vi "Main RT.vi"() -> ()   [LabVIEW 2014]
uses:
  Controls/RT State.ctl
  Controls/Current Limit Parameters.ctl
  Controls/ES System Data.ctl
  Controls/StringSelector.ctl
  Controls/FPGA Data.ctl
  Controls/ES String Array.ctl
  Controls/ES String Data.ctl
  Controls/PC Data.ctl
  Controls/MicroZed Config Op Mode.ctl
  Controls/MicroZed Config.ctl
  Controls/Gen Data.ctl
  Controls/Current Limit Output.ctl
  <vilib>/Modbus/subvis/Modbus API/Modbus API.lvclass/Modbus API.ctl
  <vilib>/Modbus/subvis/Transmission Data Unit (ADU)/Transmission Data Unit/Transmission Data Unit.lvclass/Transmission Data Unit.ctl
  <vilib>/Modbus/master/Set Unit ID.vi
  <vilib>/Modbus/master/Data Access/Unit ID/Set Unit ID Property.vi
  <vilib>/Modbus/subvis/Transmission Data Unit (ADU)/Transmission Data Unit/Data Access/Unit ID/Write Unit ID.vi
  <vilib>/Modbus/subvis/Modbus API/Read Transmission Data Unit.vi
  <vilib>/Modbus/subvis/Modbus API/Write Transmission Data Unit.vi
  <vilib>/FPGAPlugInAG/cRIO-9068/niLvFpga_Open_cRIO-9068.vi
  <vilib>/rvi/interface/common/dynamic/niFpgaDynamicAddResources.vi
  <vilib>/FPGAPlugInAG/Dynamic/niLvFpga_Reset_Dynamic.vi
  <vilib>/FPGAPlugInAG/Dynamic/niLvFpga_Run_Dynamic.vi
  <vilib>/Utility/error.llb/Error Cluster From Error Code.vi
  <vilib>/rvi/errors/niLvFpgaAdjustHostInterfaceError.vi
  <vilib>/Modbus/master/Create Master Instance.vi
  <vilib>/Modbus/master/Create Master Instance (TCP).vi
  <vilib>/Modbus/master/Set Timeouts.vi
  GenErrorParse.vi
  32Bit Two Complement.vi
  16Bit Two Complement.vi
  <vilib>/FPGAPlugInAG/Dynamic/niLvFpga_Close_Dynamic.vi
  <vilib>/rvi/interface/nirviOpenFPGA/nirviOpenFPGA.xnode
  Builds/FPGA Bitfiles/FPGA NIGHTVISION.lvbitx
  <vilib>/rvi/interface/nirviMethod/nirviMethod.xnode
  <vilib>/rvi/interface/nirviReadWriteControl/nirviReadWriteControl.xnode
  <vilib>/Modbus/master/Modbus Master.lvclass
  <vilib>/Modbus/subvis/Transmission Data Unit (ADU)/Transmission Data Unit/Transmission Data Unit.lvclass
  <vilib>/rvi/interface/nirviCloseFPGA/nirviCloseFPGA.xnode
  RT Watchdog/RT Watchdog.lvlib
  NiFpgaLv.dll
  <vilib>/rvi/interface/Simulation/niFpgaSimulationCallBeginRW.vi
  <vilib>/ptbypt/NI_PtbyPt.lvlib
panel:
  in  "PC CMD":bool=TRUE
  out "Charge Max SOC":sgl=55.0
  out "HVAC FB":bool
  out "HVAC CMD":bool=TRUE
  out "Contactor CMD FB":bool[](array[boolean])
  out "ES Cycle Count":dbl
  out "Write Data":string[](array[string])
  out "Read Data":string[](array[string])
  in  "Manual OLP":T1 {"Min Cell Voltage Actual Value" format="%#.2f"; "Max Cell Voltage Actual Value" format="%#.2f"}
  in  "Override?":bool
  out "First String Index":i32
  out "PC Count":i32
  out "Gen East Count":i32
  out "Gen West Count":i32
  out "ES Count":i32
  out "Generator ON East":bool=TRUE
  out "Generator ON West":bool=TRUE
  out "Gen Active":T2={"Warning"=FALSE, "System Fault"=FALSE, "Com Fault"=TRUE, "Alarms"=[], "ControllerMode"=0, "ActivePower(W)"=0, "ReactivePower(VAR)"=0, "PowerFactor"=0.0, "RunHours(hr)"=0.0, "Freq(Hz)"=0.0, "BattVoltage(V)"=0.0, "ApparentPower(VA)"=0, "FuelRate(L/H)"=0.0, "TotalFuel(L)"=0, "IsRunning"=FALSE} {"TotalFuel(L)" format="%.2f"; "FuelRate(L/H)" format="%.2f"; "ApparentPower(VA)" format="%.2f"; "BattVoltage(V)" format="%.2f"; "Freq(Hz)" format="%.2f"; "RunHours(hr)" format="%.2f"; "PowerFactor" format="%.2f"; "ReactivePower(VAR)" format="%.2f"; "ActivePower(W)" format="%.2f"}
  out "Gen Data East":T2={"Warning"=FALSE, "System Fault"=FALSE, "Com Fault"=TRUE, "Alarms"=[], "ControllerMode"=0, "ActivePower(W)"=0, "ReactivePower(VAR)"=0, "PowerFactor"=0.0, "RunHours(hr)"=0.0, "Freq(Hz)"=0.0, "BattVoltage(V)"=0.0, "ApparentPower(VA)"=0, "FuelRate(L/H)"=0.0, "TotalFuel(L)"=0, "IsRunning"=FALSE} {"TotalFuel(L)" format="%.2f"; "FuelRate(L/H)" format="%.2f"; "ApparentPower(VA)" format="%.2f"; "BattVoltage(V)" format="%.2f"; "Freq(Hz)" format="%.2f"; "RunHours(hr)" format="%.2f"; "PowerFactor" format="%.2f"; "ReactivePower(VAR)" format="%.2f"; "ActivePower(W)" format="%.2f"}
  out "Gen Data West":T2={"Warning"=FALSE, "System Fault"=FALSE, "Com Fault"=TRUE, "Alarms"=[], "ControllerMode"=0, "ActivePower(W)"=0, "ReactivePower(VAR)"=0, "PowerFactor"=0.0, "RunHours(hr)"=0.0, "Freq(Hz)"=0.0, "BattVoltage(V)"=0.0, "ApparentPower(VA)"=0, "FuelRate(L/H)"=0.0, "TotalFuel(L)"=0, "IsRunning"=FALSE} {"TotalFuel(L)" format="%.2f"; "FuelRate(L/H)" format="%.2f"; "ApparentPower(VA)" format="%.2f"; "BattVoltage(V)" format="%.2f"; "Freq(Hz)" format="%.2f"; "RunHours(hr)" format="%.2f"; "PowerFactor" format="%.2f"; "ReactivePower(VAR)" format="%.2f"; "ActivePower(W)" format="%.2f"}
  in  "Genset On":bool=TRUE
  out "Current Limit Output":T3
  in  "Automatic Start":bool
  in  "Clear Error":bool
  in  "PV Breaker":bool
  in  "SSG Breaker":bool
  in  "PC Config":T4={"AC Voltage SP"=0.0, "AC Current SP"=0.0, "Frequency SP"=60.0, "DC Voltage SP"=450.0, "Op Mode SP"=enum."Shutdown (Reset)", "Clear Faults SP"=0} {"Clear Faults SP" format="%01x"; "DC Voltage SP" min=300 max=550 format="%2.1f"; "Frequency SP" min=45 max=65 format="%2.1f"; "AC Current SP" min=-500 max=500 format="%2.1f"; "AC Voltage SP" min=0 max=132 format="%2.1f"}
  out "PC Data":T6={"AC Voltage- L1"=0.0, "AC Voltage - L2"=0.0, "AC Current - L1"=0.0, "AC Current - L2"=0.0, "Neutral Current"=0.0, "Temperature"=0.0, "AC Frequency"=0.0, "DC Voltage"=0.0, "AC Voltage SP"=0.0, "AC Current SP"=0.0, "Frequency SP"=0.0, "Op Mode SP"=enum."Shutdown (Reset)", "Clear Faults SP"=0, "PC Com Fault"=TRUE, "PC Fault"=FALSE, "DC Voltage SP"=0.0, "OP Mode FB"=enum."Shutdown (Reset)", "Contactor FB"=0, "Faults 1"=0, "Alarms 1"=0, "Faults 2"=0, "Alarms 2"=0, "PC Alarm"=FALSE, "Version"=0} {"Alarms 2" format="%016b"; "Faults 2" format="%016b"; "Alarms 1" format="%016b"; "Faults 1" format="%016b"; "Contactor FB" format="%.0b"; "DC Voltage SP" format="%2.1f"; "Clear Faults SP" format="%.0b"; "Neutral Current" format="%2.1f"; "AC Current - L2" format="%2.1f"; "AC Voltage - L2" format="%2.1f"; "Temperature" format="%2.1f"; "DC Voltage" format="%2.1f"; "AC Current SP" format="%2.1f"; "AC Voltage SP" format="%2.1f"; "Frequency SP" format="%2.1f"; "AC Frequency" format="%2.1f"; "AC Current - L1" format="%2.1f"; "AC Voltage- L1" format="%2.1f"}
  in  "ES ON Array":bool[](array[boolean])
  out "ES String Data":T7
  out "FPGA Data":T9 {"SSG Active Current" format="%2.1f"; "PV Reactive Power (L1)" format="%2.1f"; "PV Reactive Power (L2)" format="%2.1f"; "PV Total Reactive Power" format="%2.1f"; "Gen Reactive Power (L1)" format="%2.1f"; "Gen Reactive Power (L2)" format="%2.1f"; "Gen Total Reactive Power" format="%2.1f"; "SSG Reactive Power (L1)" format="%2.1f"; "SSG Reactive Power (L2)" format="%2.1f"; "SSG Total Reactive Power" format="%2.1f"; "PV Total Current" format="%2.1f"; "PV Total Voltage" format="%2.1f"; "PV Active Power (L1)" format="%2.1f"; "PV Active Power (L2)" format="%2.1f"; "PV App Power (L1)" format="%2.1f"; "PV App Power (L2)" format="%2.1f"; "PV Total Active Power" format="%2.1f"; "PV Total App Power" format="%2.1f"; "PV Arms (L1)" format="%2.1f"; "PV Arms (L2)" format="%2.1f"; "PV Vrms (L1)" format="%2.1f"; "PV Vrms (L2)" format="%2.1f"; "Gen Total Current" format="%2.1f"; "SSG Total Current" format="%2.1f"; "Gen Total Voltage" format="%2.1f"; "SSG Total Voltage" format="%2.1f"; "Gen Active Power (L1)" format="%2.1f"; "Gen Active Power (L2)" format="%2.1f"; "SSG Active Power (L1)" format="%2.1f"; "SSG Active Power (L2)" format="%2.1f"; "Gen App Power (L1)" format="%2.1f"; "Gen App Power (L2)" format="%2.1f"; "SSG App Power (L1)" format="%2.1f"; "SSG App Power (L2)" format="%2.1f"; "Gen Total Active Power" format="%2.1f"; "Gen Total App Power" format="%2.1f"; "Gen Arms (L1)" format="%2.1f"; "Gen Arms (L2)" format="%2.1f"; "Gen Vrms (L1)" format="%2.1f"; "Gen Vrms (L2)" format="%2.1f"; "SSG Total Active Power" format="%2.1f"; "SSG Total App Power" format="%2.1f"; "SSG Arms (L1)" format="%2.1f"; "SSG Arms (L2)" format="%2.1f"; "SSG Vrms (L1)" format="%2.1f"; "SSG Vrms (L2)" format="%2.1f"}
  out "ES System Data":T10={"Voltage"=0.0, "Current"=0.0, "SOC Avg"=0.0, "Faults"=0, "Alarms"=0, "# Strings"=0, "Max Temp"=0, "Min Temp"=0, "Max Cell Voltage"=0.0, "Min Cell Voltage"=0.0, "Energy Capacity"=0.0, "Energy Remaining"=0.0, "SOC Min"=0.0, "SOC Max"=0.0, "ES Fault"=FALSE, "String Select"=enum."3 Strings", "ES Com Fault"=TRUE, "SOH Avg"=0.0}
  out "Current Limit Parameters":T1 {"Min Cell Voltage Actual Value" format="%#.2f"; "Max Cell Voltage Actual Value" format="%#.2f"}
  out "Real Time State":T12
  in  "stop":bool
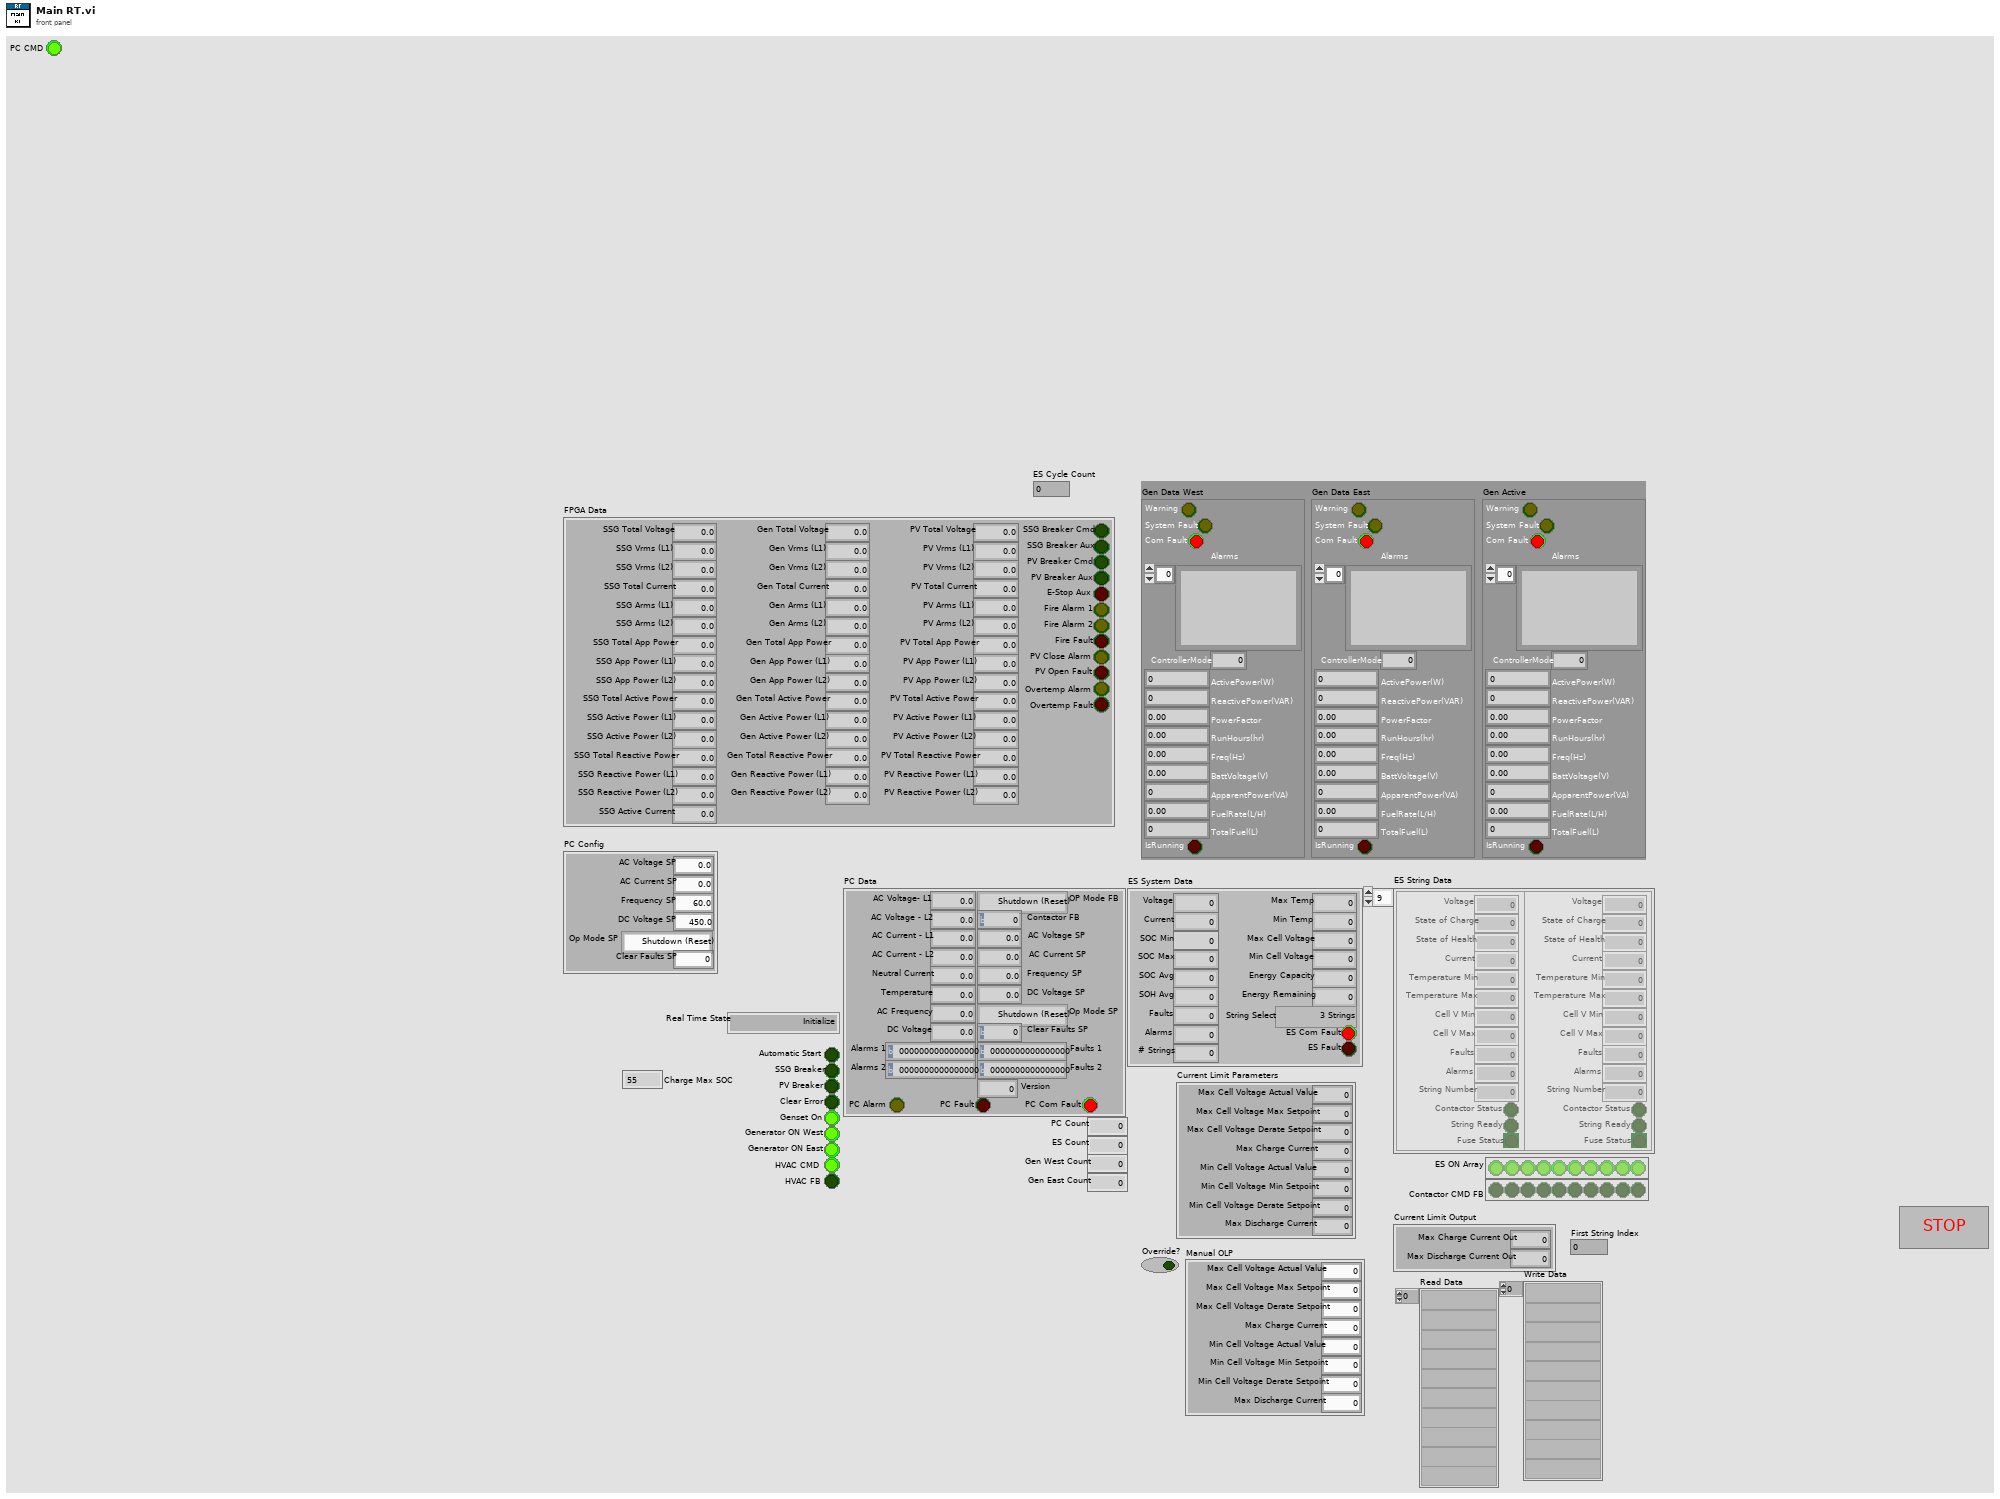
[diagram p1: front panel]
types:
  T1 = typedef "Current Limit Parameters.ctl" = cluster{"Max Cell Voltage Max Setpoint":dbl, "Max Cell Voltage Actual Value":dbl, "Max Cell Voltage Derate Setpoint":dbl, "Max Charge Current":dbl, "Min Cell Voltage Min Setpoint":dbl, "Min Cell Voltage Actual Value":dbl, "Min Cell Voltage Derate Setpoint":dbl, "Max Discharge Current":dbl}
  T2 = typedef "Gen Data.ctl" = cluster{"Warning":bool, "System Fault":bool, "Com Fault":bool, "Alarms":string[], "ControllerMode":u16, "ActivePower(W)":i32, "ReactivePower(VAR)":i32, "PowerFactor":dbl, "RunHours(hr)":dbl, "Freq(Hz)":dbl, "BattVoltage(V)":dbl, "ApparentPower(VA)":i32, "FuelRate(L/H)":dbl, "TotalFuel(L)":u32, "IsRunning":bool}
  T3 = typedef "Current Limit Output.ctl" = cluster{"Max Charge Current Out":dbl, "Max Discharge Current Out":dbl}
  T4 = typedef "MicroZed Config.ctl" = cluster{"AC Voltage SP":sgl, "AC Current SP":sgl, "Frequency SP":sgl, "DC Voltage SP":sgl, "Op Mode SP":T5, "Clear Faults SP":i16}
  T5 = typedef "MicroZed Config Op Mode.ctl" = enum16{"Shutdown (Reset)", "Startup", "Idle", "Voltage Mode", "Current Mode", "Fault", "OL Voltage (Debug)", "No Data"}
  T6 = typedef "PC Data.ctl" = cluster{"AC Voltage- L1":dbl, "AC Voltage - L2":dbl, "AC Current - L1":dbl, "AC Current - L2":dbl, "Neutral Current":dbl, "Temperature":dbl, "AC Frequency":dbl, "DC Voltage":dbl, "AC Voltage SP":dbl, "AC Current SP":dbl, "Frequency SP":dbl, "Op Mode SP":T5, "Clear Faults SP":u16, "PC Com Fault":bool, "PC Fault":bool, "DC Voltage SP":dbl, "OP Mode FB":T5, "Contactor FB":u16, "Faults 1":u16, "Alarms 1":u16, "Faults 2":u16, "Alarms 2":u16, "PC Alarm":bool, "Version":u16}
  T7 = typedef "ES String Array.ctl" = T8[]
  T8 = typedef "ES String Data.ctl" = cluster{"Voltage":sgl, "State of Charge":sgl, "Current":sgl, "Temperature Min":i16, "Temperature Max":i16, "Faults":u16, "Alarms":u16, "String Number":u16, "Contactor Status":bool, "String Ready":bool, "Fuse Status":bool, "Cell V Max":dbl, "Cell V Min":dbl, "State of Health":sgl}
  T9 = typedef "FPGA Data.ctl" = cluster{"Gen Total Voltage":dbl, "Gen Vrms (L1)":dbl, "Gen Vrms (L2)":dbl, "Gen Total Current":dbl, "Gen Arms (L1)":dbl, "Gen Arms (L2)":dbl, "Gen Total App Power":dbl, "Gen App Power (L1)":dbl, "Gen App Power (L2)":dbl, "Gen Total Active Power":dbl, "Gen Active Power (L1)":dbl, "Gen Active Power (L2)":dbl, "Gen Total Reactive Power":dbl, "Gen Reactive Power (L1)":dbl, "Gen Reactive Power (L2)":dbl, "SSG Total Voltage":dbl, "SSG Vrms (L1)":dbl, "SSG Vrms (L2)":dbl, "SSG Total Current":dbl, "SSG Arms (L1)":dbl, "SSG Arms (L2)":dbl, "SSG Total App Power":dbl, "SSG App Power (L1)":dbl, "SSG App Power (L2)":dbl, "SSG Total Active Power":dbl, "SSG Active Power (L1)":dbl, "SSG Active Power (L2)":dbl, "SSG Total Reactive Power":dbl, "SSG Reactive Power (L1)":dbl, "SSG Reactive Power (L2)":dbl, "PV Total Voltage":dbl, "PV Vrms (L1)":dbl, "PV Vrms (L2)":dbl, "PV Total Current":dbl, "PV Arms (L1)":dbl, "PV Arms (L2)":dbl, "PV Total App Power":dbl, "PV App Power (L1)":dbl, "PV App Power (L2)":dbl, "PV Total Active Power":dbl, "PV Active Power (L1)":dbl, "PV Active Power (L2)":dbl, "PV Total Reactive Power":dbl, "PV Reactive Power (L1)":dbl, "PV Reactive Power (L2)":dbl, "SSG Breaker Cmd":bool, "SSG Breaker Aux":bool, "PV Breaker Cmd":bool, "PV Breaker Aux":bool, "E-Stop Aux":bool, "Fire Alarm 1":bool, "Fire Alarm 2":bool, "Fire Fault":bool, "PV Close Alarm":bool, "SSG Active Current":dbl, "Overtemp Alarm":bool, "Overtemp Fault":bool, "PV Open Fault":bool}
  T10 = typedef "ES System Data.ctl" = cluster{"Voltage":sgl, "Current":sgl, "SOC Avg":sgl, "Faults":u16, "Alarms":u16, "# Strings":u16, "Max Temp":i16, "Min Temp":i16, "Max Cell Voltage":sgl, "Min Cell Voltage":sgl, "Energy Capacity":sgl, "Energy Remaining":sgl, "SOC Min":sgl, "SOC Max":sgl, "ES Fault":bool, "String Select":T11, "ES Com Fault":bool, "SOH Avg":sgl}
  T11 = typedef "StringSelector.ctl" = enum16{"1 String (1)", "1 String (2)", "1 String (3)", "2 Strings (1 2)", "2 Strings (2 3)", "2 Strings (1 3)", "3 Strings"}
  T12 = typedef "RT State.ctl" = enum16{"Initialize", "Ready", "Startup 1 - Start Genset", "Startup 2 - Start Inverter", "Startup 3 - Battery Match", "SpotGen - Start", "SpotGen - Charge", "SpotGen - Desync", "SpotGen - Discharge", "SpotGen - Sync", "Shutdown", "INVALID STATE"}
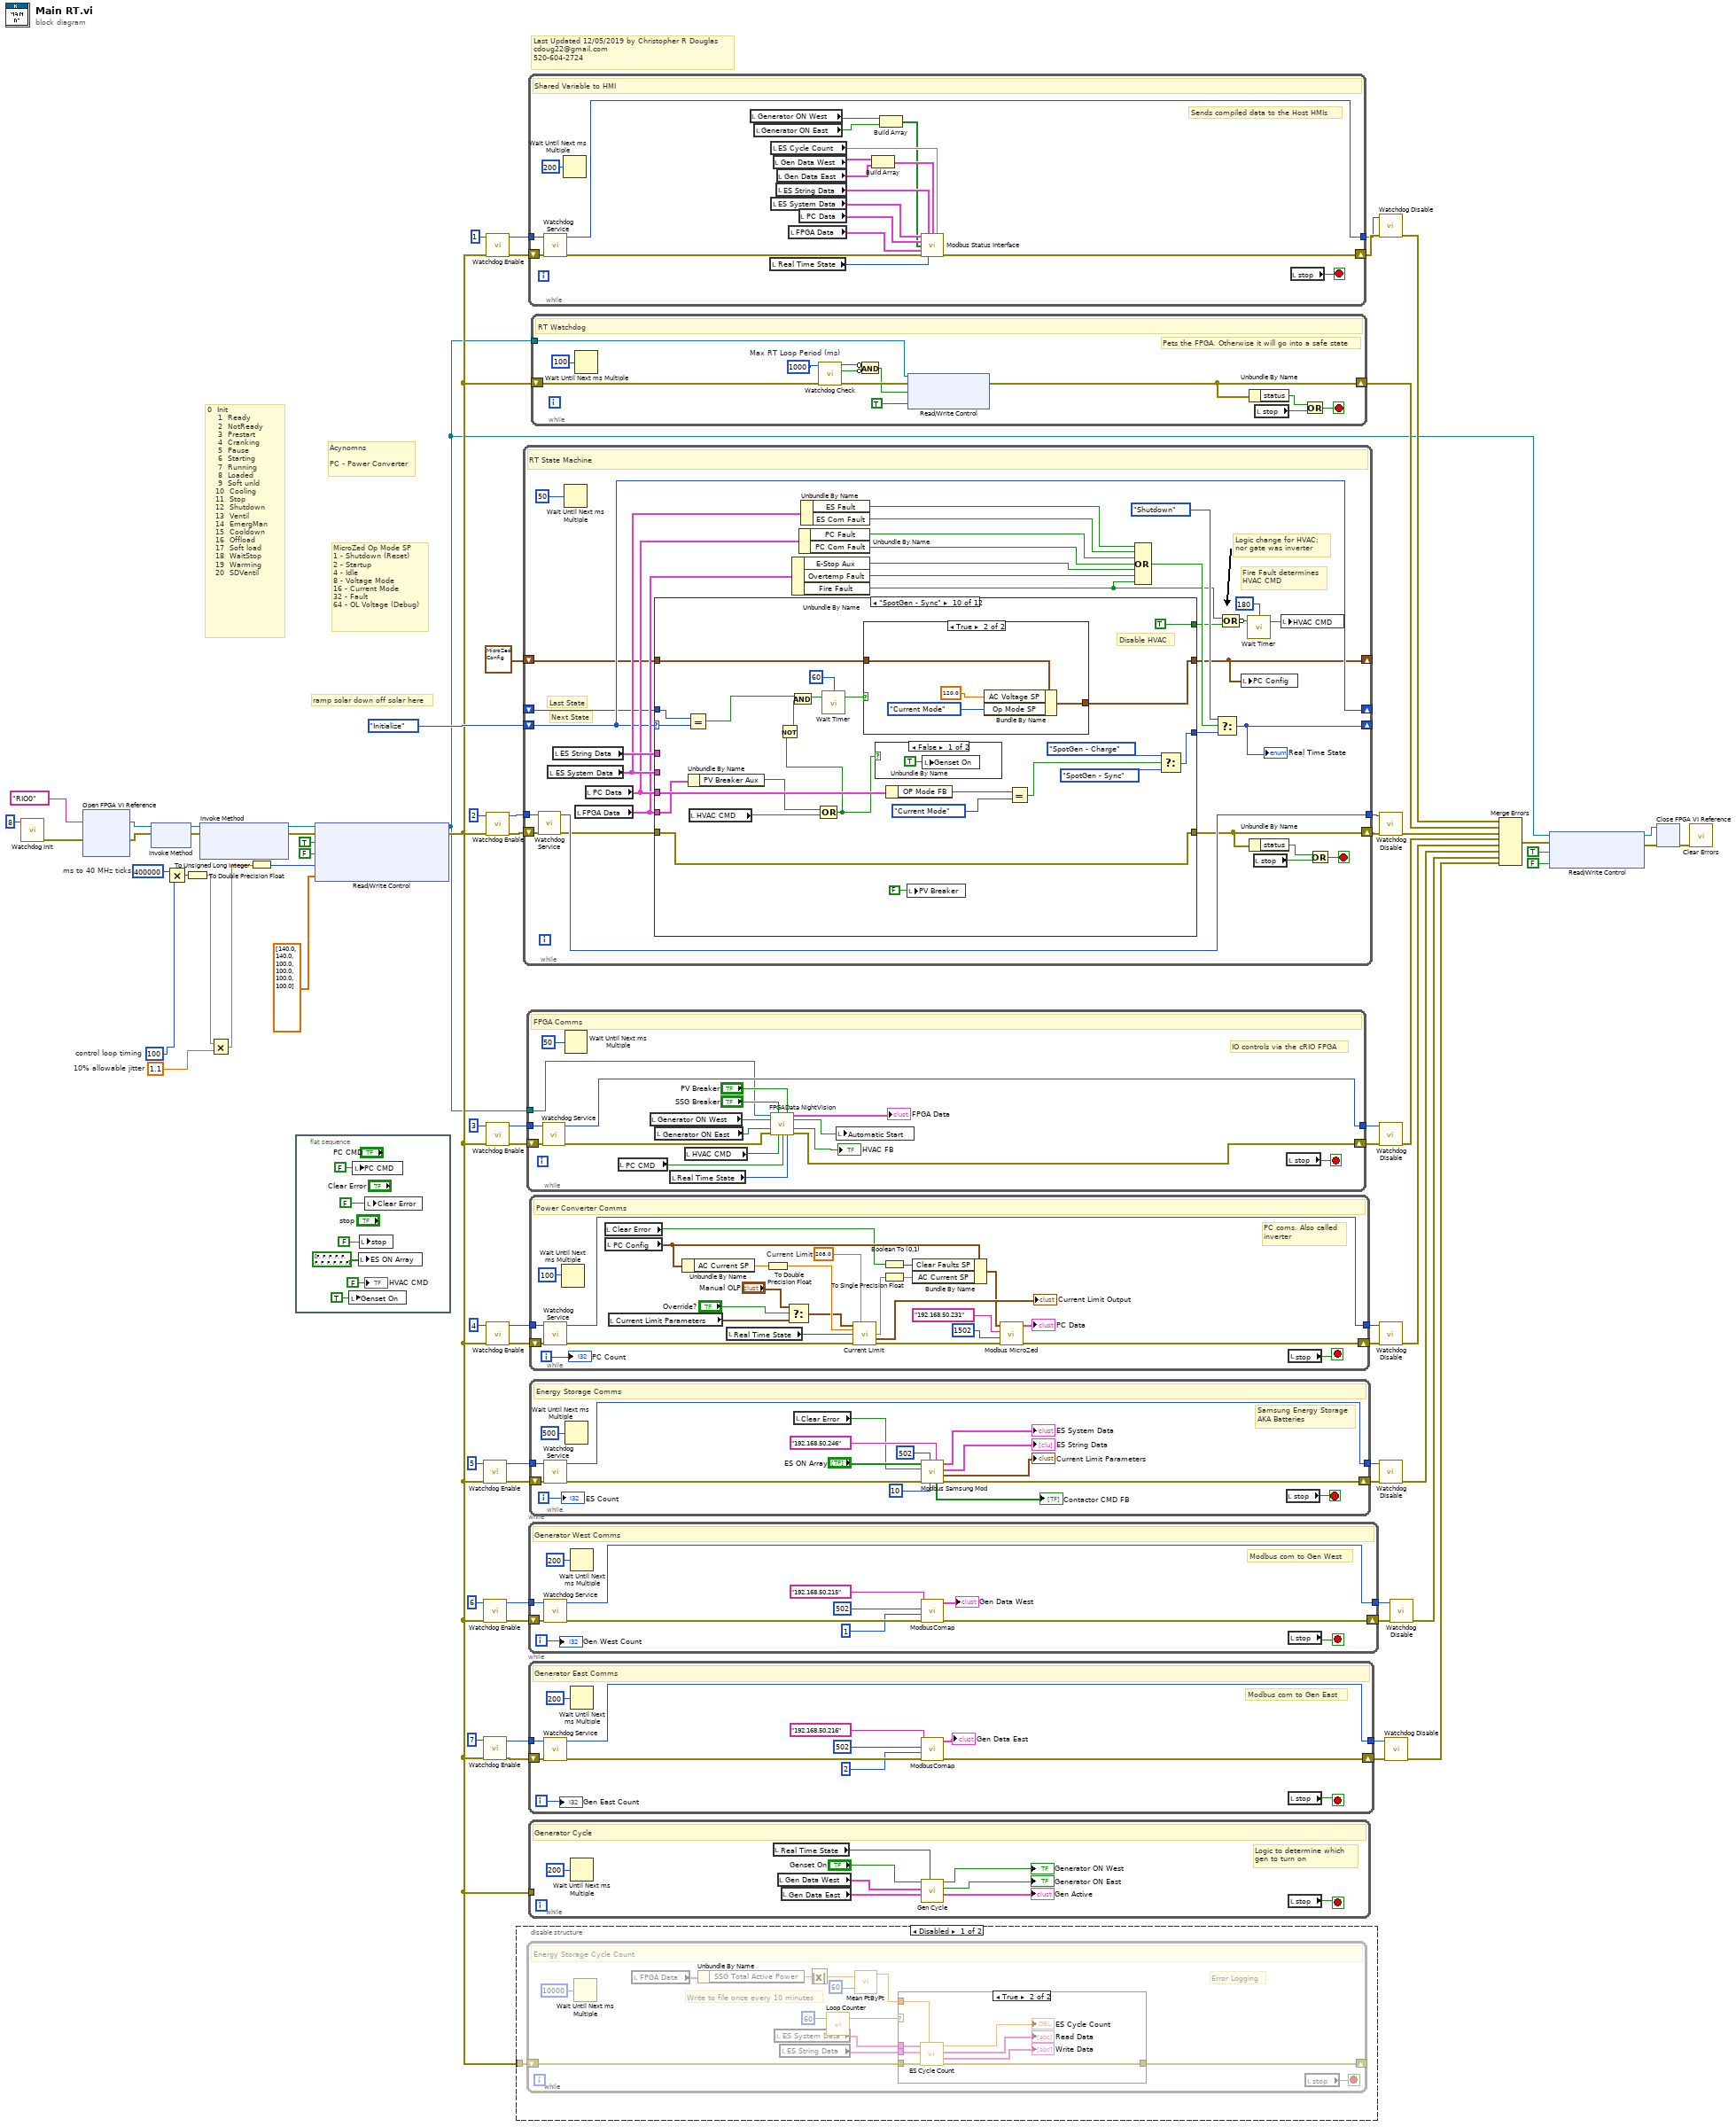
[diagram p0: block diagram]
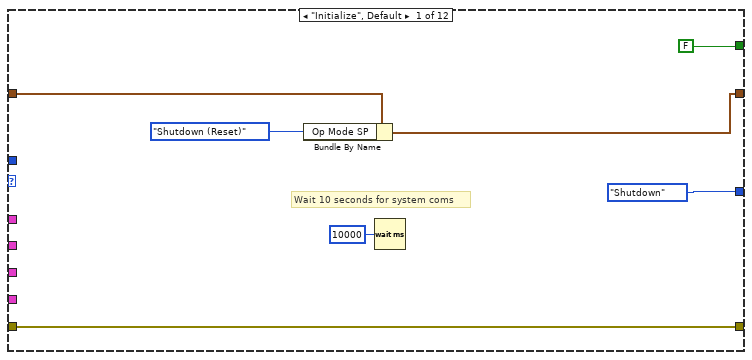
[diagram p4: hidden frame]
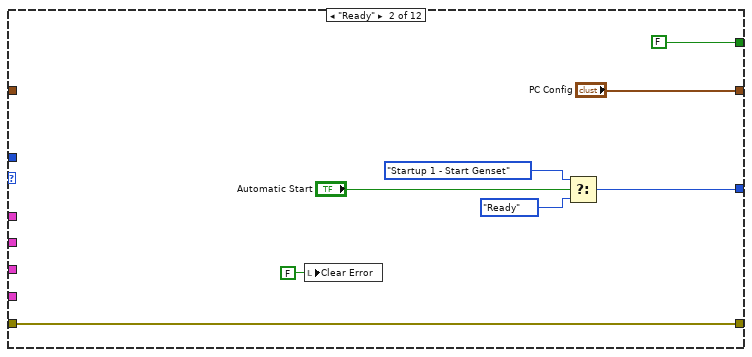
[diagram p5: hidden frame]
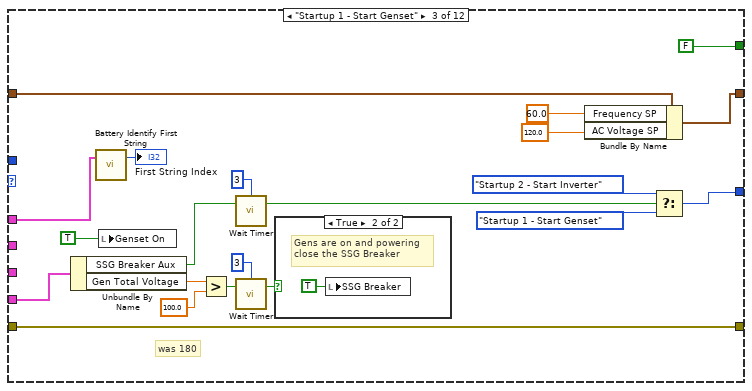
[diagram p6: hidden frame]
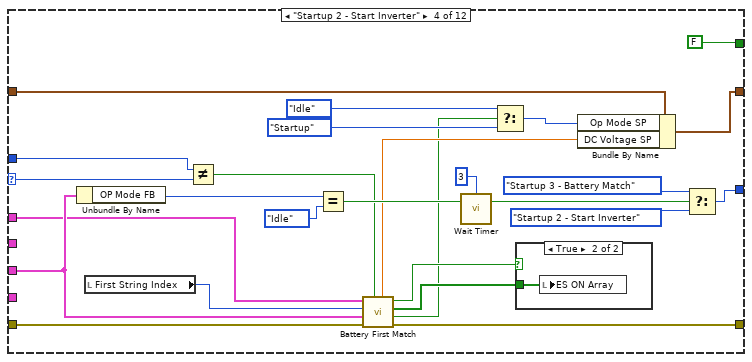
[diagram p8: hidden frame]
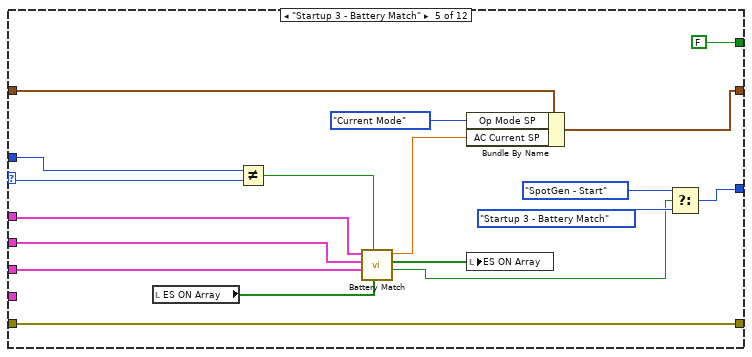
[diagram p10: hidden frame]
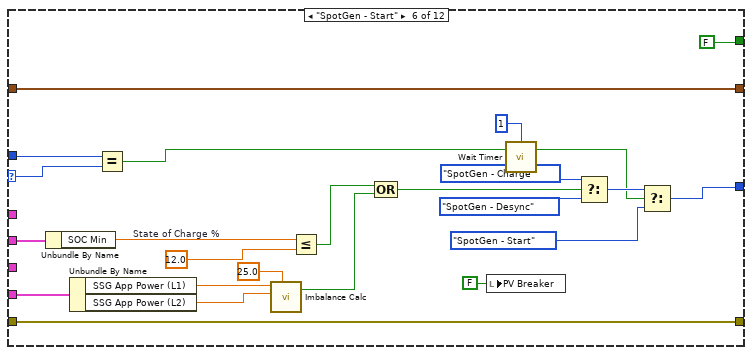
[diagram p11: hidden frame]
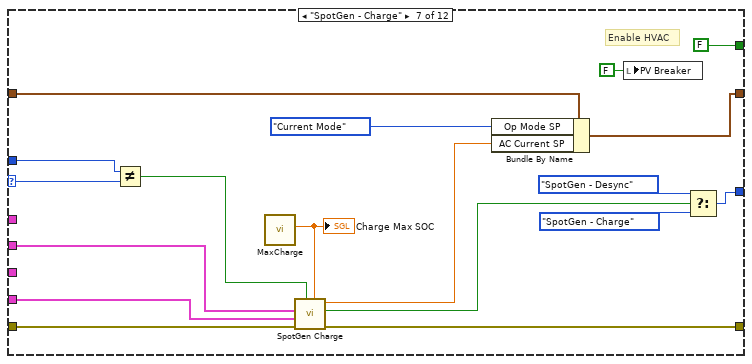
[diagram p12: hidden frame]
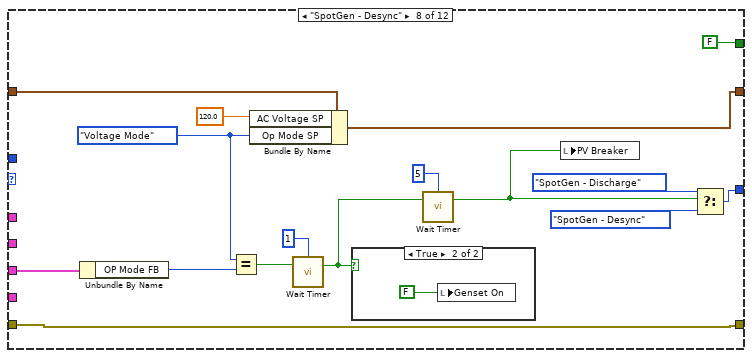
[diagram p13: hidden frame]
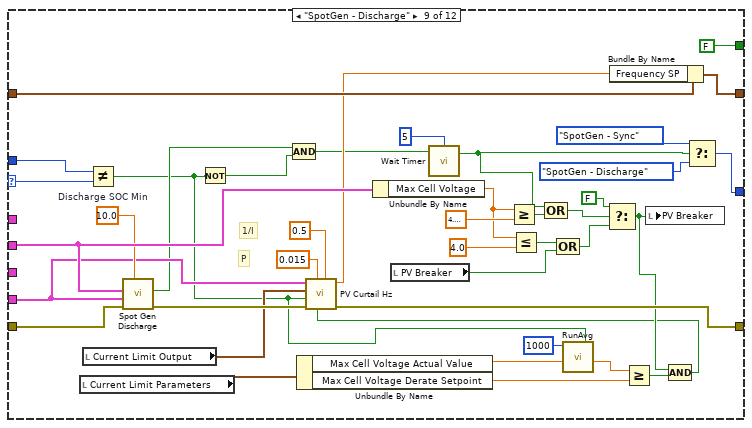
[diagram p15: hidden frame]
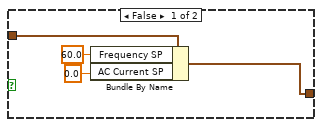
[diagram p17: hidden frame]
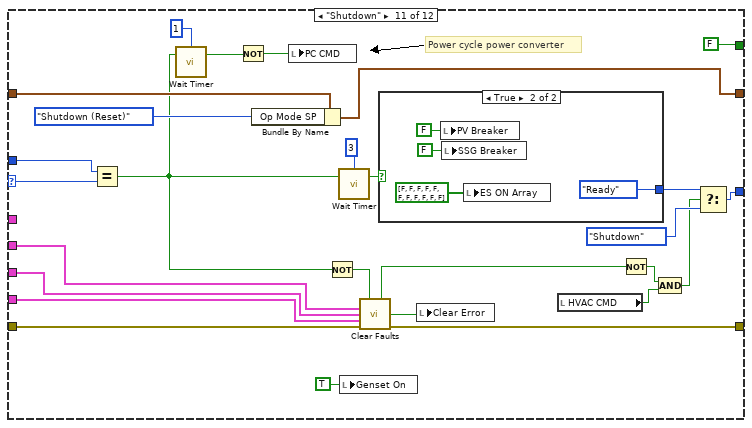
[diagram p18: hidden frame]
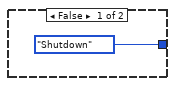
[diagram p19: hidden frame]
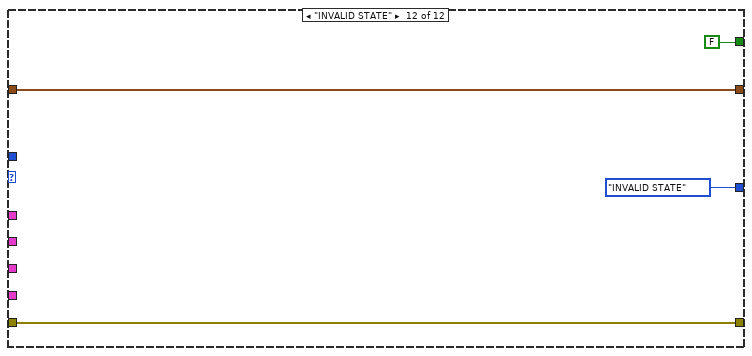
[diagram p20: hidden frame]
diagram:
  w52 = i64 100  # control loop timing
  w55 = 1.1  # 10% allowable jitter
  w57 = i64 400000  # ms to 40 MHz ticks
  # "Acynomns\n\nPC - Power Converter"
  # "Last Updated 12/05/2019 by Christopher R Douglas \ncdoug22@gmail.com\n520-604-2724"
  # "0  Init          \n    1  Ready         \n    2  NotReady      \n    3  Prestart      \n    4  Cranking      \n    5  Pause         \n    6  Starting      \n    7  Running       \n    8  Loaded        \n    9  Soft unld     \n   10  Cooling       \n   11  Stop          \n   12  Shutdown      \n   13  Ventil        \n   14  EmergMan      \n   15  Cooldown      \n   16  Offload       \n   17  Soft load     \n   18  WaitStop      \n   19  Warming       \n   20  SDVentil"
  # "ramp solar down off solar here"
  # "MicroZed Op Mode SP\n1 - Shutdown (Reset)\n2 - Startup\n4 - Idle\n8 - Voltage Mode\n16 - Current Mode\n32 - Fault\n64 - OL Voltage (Debug)"
  n1 = call "Watchdog Init.vi"("Number of Watchdogs"=8) -> ("error out"=w7:errorcluster)  [unwired: 10 in]
  n2 = xnode "Open FPGA VI Reference"("error in"=w7, "resource name"=tag "RIO0") -> ("FPGA VI Reference Out"=w2:refnum<k20>, "error out"=w4:errorcluster)
  n3 = xnode "Invoke Method"("FPGA VI Reference In"=w2, "error in"=w4) -> ("FPGA VI Reference Out"=w6:refnum<k20>, "error out"=w5:errorcluster)
  n4 = Multiply(x=w57, y=w52) -> (x*y=w56:i64)
  n5 = To Double Precision Float(number=w56) -> (double precision float=w51:dbl)
  n6 = xnode "Invoke Method"("FPGA VI Reference In"=w6, "error in"=w5) -> ("FPGA VI Reference Out"=w49:refnum<k20>, "error out"=w50:errorcluster)  [unwired: 1 in]
  n7 = Multiply(x=w51, y=w55) -> (x*y=w54:dbl)
  n8 = To Unsigned Long Integer(number=w54) -> (unsigned 32bit integer=w48:u32)
  n9 = flat-sequence {
    frame #0 {
      n10 = local write "Genset On"(TRUE ("Genset On")) -> ()
      n11 = local write "PC CMD"(FALSE ("PC CMD")) -> ()
      n12 = local write "ES ON Array"(bool[] [FALSE, FALSE, FALSE, FALSE, FALSE, FALSE, FALSE, FALSE, FALSE, FALSE, FALSE] ("ES ON Array")) -> ()
      n13 = local write "stop"(FALSE ("stop")) -> ()
      n14 = local write "Clear Error"(FALSE ("Clear Error")) -> ()
      "HVAC CMD" <- FALSE ("HVAC CMD")
    }
  }
  n15 = xnode "Read/Write Control"("FPGA VI Reference In"=w49, "error in"=w50, "Enable RT Watchdog"=TRUE, "RT Reset on Watchdog Failure?"=FALSE, "RT Timeout Period (ticks)"=w48, "CT Scales"=sgl[] [140.0, 140.0, 100.0, 100.0, 100.0, 100.0] ("CT Scale")) -> ("FPGA VI Reference Out"=w1:refnum<k20>, "error out"=w29:errorcluster)
  n16 = call "Watchdog Enable.vi"("error in (no error)"=w29, "Watchdog Index"=5) -> ("error out"=w37:errorcluster, "Watchdog Index Out"=w35:i32)  [unwired: 8 in]
  n17 = call "Watchdog Enable.vi"("error in (no error)"=w29, "Watchdog Index"=6) -> ("error out"=w12:errorcluster, "Watchdog Index Out"=w10:i32)  [unwired: 8 in]
  n18 = call "Watchdog Enable.vi"("error in (no error)"=w29, "Watchdog Index"=7) -> ("error out"=w27:errorcluster, "Watchdog Index Out"=w24:i32)  [unwired: 8 in]
  n19 = call "Watchdog Enable.vi"("error in (no error)"=w29, "Watchdog Index"=1) -> ("error out"=w40:errorcluster, "Watchdog Index Out"=w38:i32)  [unwired: 8 in]
  n20 = call "Watchdog Enable.vi"("error in (no error)"=w29, "Watchdog Index"=2) -> ("error out"=w65:errorcluster, "Watchdog Index Out"=w63:i32)  [unwired: 8 in]
  n21 = call "Watchdog Enable.vi"("error in (no error)"=w29, "Watchdog Index"=3) -> ("error out"=w44:errorcluster, "Watchdog Index Out"=w43:i32)  [unwired: 8 in]
  n22 = call "Watchdog Enable.vi"("error in (no error)"=w29, "Watchdog Index"=4) -> ("error out"=w66:errorcluster, "Watchdog Index Out"=w67:i32)  [unwired: 8 in]
  n23 = disable-structure shown="Disabled" {
    disable-tunnel: w29 -> [w79 _]
    frame Disabled {
      n24 = while {
        shift-right: [w90] -> _
        shift-left: w79 -> [w91]
        stop <- w89 stop-if-true
        # "Error Logging"
        # "Write to file once every 10 minutes"
        # "Energy Storage Cycle Count"
        n25 = Wait Until Next ms Multiple(millisecond multiple=u32 10000 ("milliseconds to wait")) -> ()  [unwired: 1 out]
        n26 = local read "FPGA Data"() -> (w86:T9)
        n27 = Unbundle By Name(w86) -> ("SSG Total Active Power"=w87:dbl)
        n28 = local read "ES System Data"() -> (w81:T10)
        n29 = local read "ES String Data"() -> (w82:T7)
        n30 = Absolute Value(x=w87) -> (abs(x)=w83:dbl)
        n31 = call "Loop Counter.vi"("Time to Wait A"=u8 60) -> ("Time Expired A"=w80:bool)  [unwired: 2 in]
        n32 = call <vilib>:"Mean PtByPt.vi"("x"=w83, "sample length"=60) -> ("mean"=w85:dbl)  [unwired: 2 in, 1 out]
        n33 = case shown="True" w80 {
          tunnel: w91 -> [w93 w101]
          tunnel: [w93 w100] -> w90
          tunnel: w85 -> [_ w99]
          tunnel: w82 -> [_ w98]
          tunnel: w81 -> [_ w97]
          frame False {
          }
          frame True {
            n34 = call "ES Cycle Count.vi"("SSG Average Total Active Power"=w99, "Error In"=w101, "ES String Data"=w98, "ES System Data"=w97) -> ("error out"=w100:errorcluster, "Write Data"=→"Write Data":string[], "Read Data"=→"Read Data":string[], "# cycles"=→"ES Cycle Count":dbl)  [unwired: 4 in]
          }
        }
        n35 = local read "stop"() -> (w89:bool)
      }
    }
    frame Enabled {
    }
  }
  n36 = while "System State Machine" {
    tunnel: w63 -> [w132]
    tunnel: [w125] -> w20
    shift-right: [w121] -> _
    shift-left: RT_State."Initialize" -> [w118]
    shift-right: [w105] -> w21
    shift-left: w65 -> [w133]
    shift-right: [w107] -> _
    shift-left: T4 {"AC Voltage SP"=0.0, "AC Current SP"=0.0, "Frequency SP"=60.0, "DC Voltage SP"=450.0, "Op Mode SP"=enum."Shutdown (Reset)", "Clear Faults SP"=0} ("PC Config") -> [w108]
    shift-right: [w118] -> _
    shift-left: _ -> [w117]
    stop <- w128 stop-if-true
    # "Logic change for HVAC:\nnor gate was inverter"
    # "Fire Fault determines \nHVAC CMD"
    # "Next State"
    # "Last State"
    # "RT State Machine"
    n37 = call "Watchdog Service.vi"("error in (no error)"=w133, "Watchdog Index"=w132) -> ("error out"=w106:errorcluster, "Watchdog Index Out"=w125:i32)  [unwired: 8 in]
    n38 = local read "ES System Data"() -> (w123:T10)
    n39 = local read "ES String Data"() -> (w124:T7)
    n40 = Wait Until Next ms Multiple(millisecond multiple=u32 50 ("milliseconds to wait")) -> ()  [unwired: 1 out]
    n41 = local read "FPGA Data"() -> (w119:T9)
    n42 = local read "PC Data"() -> (w122:T6)
    n43 = case shown="\"SpotGen - Sync\"" w118 {
      selector: w118 -> [_ _ _ w177 w202 w236 w248 _ w308 w324 w370 _]
      tunnel: [RT_State."Shutdown" w146 w162 w194 w214 w235 w255 w271 w314 w336 w366 RT_State."INVALID STATE" ("Real Time State")] -> w131
      tunnel: w122 -> [_ _ _ w185 w211 _ _ w270 _ w335 w368 _]
      tunnel: w123 -> [_ _ _ _ w212 w239 w253 _ w307 _ w367 _]
      tunnel: w124 -> [_ _ w154 w182 w213 _ _ _ _ _ _ _]
      tunnel: w119 -> [_ _ w169 _ _ w238 w254 _ w284 w323 w369 _]
      tunnel: w117 -> [_ _ _ w178 w203 w237 w249 _ w300 w325 w371 _]
      tunnel: w108 -> [w136 _ w152 w175 w201 w218 w247 w261 w286 w328 w357 w382]
      tunnel: [w135 "PC Config" w151 w174 w200 w218 w246 w260 w299 w326 w356 w382] -> w107
      tunnel: w106 -> [w139 w142 w150 w172 w199 w217 w245 w259 w292 w322 w355 w381]
      tunnel: [w139 w142 w150 w173 w199 w217 w244 w259 w291 w322 w354 w381] -> w105
      tunnel: [FALSE FALSE FALSE FALSE FALSE FALSE FALSE FALSE FALSE TRUE FALSE FALSE] -> w102
      frame "Initialize", Default {
        # "Wait 10 seconds for system coms"
        n44 = Bundle By Name(cluster=w136, "Op Mode SP"=MicroZed_Config_Op_Mode."Shutdown (Reset)") -> (w135:T4)
        n45 = Wait (ms)(milliseconds to wait=u32 10000) -> ()  [unwired: 1 out]
      }
      frame "Ready" {
        n46 = local write "Clear Error"(FALSE ("Clear Error")) -> ()
        n47 = Select(t=RT_State."Startup 1 - Start Genset", s="Automatic Start", f=RT_State."Ready") -> (s? t:f=w146:T12)
      }
      frame "Startup 1 - Start Genset" {
        # "was 180"
        n48 = Unbundle By Name(w169) -> ("SSG Breaker Aux"=w160:bool, "Gen Total Voltage"=w168:dbl)
        n49 = call "Battery Identify First String.vi"("ES String Data"=w154) -> ("Index"=→"First String Index":i32)  [unwired: 2 in]
        n50 = local write "Genset On"(TRUE ("Genset On")) -> ()
        n51 = Greater?(x=w168, y=100.0) -> (0:w166:bool)
        n52 = call "Wait Timer.vi"("Boolean In"=w160, "Timer"=u32 3) -> ("Boolean Out"=w158:bool)  [unwired: 3 in]
        n53 = call "Wait Timer.vi"("Boolean In"=w166, "Timer"=u32 3) -> ("Boolean Out"=w161:bool)  [unwired: 3 in]
        n54 = case shown="True" w161 {
          frame False {
          }
          frame True {
            # "Gens are on and powering\nclose the SSG Breaker"
            n55 = local write "SSG Breaker"(TRUE ("SSG Breaker")) -> ()
          }
        }
        n56 = Bundle By Name(cluster=w152, "Frequency SP"=sgl 60.0, "AC Voltage SP"=sgl 120.0) -> (w151:T4)
        n57 = Select(t=RT_State."Startup 2 - Start Inverter", s=w158, f=RT_State."Startup 1 - Start Genset") -> (s? t:f=w162:T12)
      }
      frame "Startup 2 - Start Inverter" {
        n58 = Unbundle By Name(w185) -> ("OP Mode FB"=w189:T5)
        n59 = local read "First String Index"() -> (w181:i32)
        n60 = Not Equal?(x=w178, y=w177) -> (x != y?=w176:bool)
        n61 = Equal?(x=w189, y=MicroZed_Config_Op_Mode."Idle" ("Op Mode SP")) -> (x = y?=w191:bool)
        n62 = call "Battery First Match.vi"("Safety Init"=w176, "Error In"=w172, "PC Data"=w185, "String Index"=w181, "ES String Data"=w182) -> ("Error Out"=w173:errorcluster, "Contactor Closed"=w179:bool, "ES ON Array"=w184:bool[], "Close Command Sent"=w180:bool, "DC Link Command"=w183:sgl)  [unwired: 2 in]
        n63 = call "Wait Timer.vi"("Boolean In"=w191, "Timer"=u32 3) -> ("Boolean Out"=w187:bool)  [unwired: 3 in]
        n64 = Select(t=MicroZed_Config_Op_Mode."Idle" ("Op Mode SP"), s=w179, f=MicroZed_Config_Op_Mode."Startup" ("Op Mode SP")) -> (s? t:f=w186:T5)
        n65 = case shown="True" w180 {
          tunnel: w184 -> [_ w197]
          frame False {
          }
          frame True {
            n66 = local write "ES ON Array"(w197) -> ()
          }
        }
        n67 = Bundle By Name(cluster=w175, "Op Mode SP"=w186, "DC Voltage SP"=w183) -> (w174:T4)
        n68 = Select(t=RT_State."Startup 3 - Battery Match", s=w187, f=RT_State."Startup 2 - Start Inverter") -> (s? t:f=w194:T12)
      }
      frame "Startup 3 - Battery Match" {
        n69 = local read "ES ON Array"() -> (w205:bool[])
        n70 = Not Equal?(x=w203, y=w202) -> (x != y?=w204:bool)
        n71 = call "Battery Match.vi"("ES ON Array In"=w205, "Init"=w204, "PC Data"=w211, "ES System Data"=w212, "ES String Data"=w213) -> ("Matching Complete"=w209:bool, "ES ON Array Out"=w210:bool[], "Precharge Current Out"=w207:sgl)  [unwired: 3 in, 1 out]
        n72 = Bundle By Name(cluster=w201, "Op Mode SP"=MicroZed_Config_Op_Mode."Current Mode", "AC Current SP"=w207) -> (w200:T4)
        n73 = local write "ES ON Array"(w210) -> ()
        n74 = Select(t=RT_State."SpotGen - Start", s=w209, f=RT_State."Startup 3 - Battery Match") -> (s? t:f=w214:T12)
      }
      frame "SpotGen - Start" {
        w219 = sgl 12.0  # State of Charge %
        n75 = Unbundle By Name(w239) -> ("SOC Min"=w234:sgl)
        n76 = Unbundle By Name(w238) -> ("SSG App Power (L1)"=w233:dbl, "SSG App Power (L2)"=w232:dbl)
        n77 = Equal?(x=w237, y=w236) -> (x = y?=w221:bool)
        n78 = call "Imbalance Calc.vi"("A"=w233, "B"=w232, "X"=25.0) -> ("|A-B|>X?"=w229:bool)  [unwired: 3 in]
        n79 = Less Or Equal?(x=w234, y=w219) -> (x <= y?=w230:bool)
        n80 = Compound Arithmetic op=OR(w230, w229) -> (w226:bool)
        n81 = local write "PV Breaker"(FALSE ("PV Breaker")) -> ()
        n82 = call "Wait Timer.vi"("Boolean In"=w221, "Timer"=u32 1) -> ("Boolean Out"=w220:bool)  [unwired: 3 in]
        n83 = Select(t=RT_State."SpotGen - Charge", s=w226, f=RT_State."SpotGen - Desync") -> (s? t:f=w225:T12)
        n84 = Select(t=w225, s=w220, f=RT_State."SpotGen - Start") -> (s? t:f=w235:T12)
      }
      frame "SpotGen - Charge" {
        # "Enable HVAC"
        n85 = Not Equal?(x=w249, y=w248) -> (x != y?=w243:bool)
        n86 = call "MaxCharge.vi"() -> ("Max SOC"=w240:sgl)  [unwired: 11 in]
        "Charge Max SOC" <- w240
        n87 = call "SpotGen Charge.vi"("Charge Max SOC"=w240, "Init"=w243, "Error In"=w245, "FPGA Data"=w254, "ES System Data"=w253) -> ("Error Out"=w244:errorcluster, "Exit Charge Mode"=w252:bool, "Current Setpoint"=w251:dbl)  [unwired: 3 in, 1 out]
        n88 = Bundle By Name(cluster=w247, "Op Mode SP"=MicroZed_Config_Op_Mode."Current Mode", "AC Current SP"=w251) -> (w246:T4)
        n89 = local write "PV Breaker"(FALSE ("PV Breaker")) -> ()
        n90 = Select(t=RT_State."SpotGen - Desync", s=w252, f=RT_State."SpotGen - Charge") -> (s? t:f=w255:T12)
      }
      frame "SpotGen - Desync" {
        w267 = MicroZed_Config_Op_Mode."Voltage Mode" ("Op Mode SP")
        n91 = Unbundle By Name(w270) -> ("OP Mode FB"=w268:T5)
        n92 = Equal?(x=w267, y=w268) -> (x = y?=w266:bool)
        n93 = Bundle By Name(cluster=w261, "AC Voltage SP"=sgl 120.0 ("Voltage Setpoint"), "Op Mode SP"=w267) -> (w260:T4)
        n94 = call "Wait Timer.vi"("Boolean In"=w266, "Timer"=u32 1) -> ("Boolean Out"=w263:bool)  [unwired: 3 in]
        n95 = case shown="True" w263 {
          frame False {
          }
          frame True {
            n96 = local write "Genset On"(FALSE ("Genset On")) -> ()
          }
        }
        n97 = call "Wait Timer.vi"("Boolean In"=w263, "Timer"=u32 5) -> ("Boolean Out"=w262:bool)  [unwired: 3 in]
        n98 = local write "PV Breaker"(w262) -> ()
        n99 = Select(t=RT_State."SpotGen - Discharge", s=w262, f=RT_State."SpotGen - Desync") -> (s? t:f=w271:T12)
      }
      frame "SpotGen - Discharge" {
        w301 = sgl 10.0  # Discharge SOC Min
        # "P"
        # "1/I"
        n100 = local read "Current Limit Parameters"() -> (w297:T1)
        n101 = local read "Current Limit Output"() -> (w311:T3)
        n102 = Not Equal?(x=w300, y=w308) -> (x != y?=w276:bool)
        n103 = call "Spot Gen Discharge.vi"("Discharge SOC Min"=w301, "Error In"=w292, "FPGA Data"=w284, "ES System Data"=w307) -> ("Error Out"=w312:errorcluster, "Exit Discharge Mode"=w278:bool)  [unwired: 6 in]
        n104 = Not(x=w276) -> (.not. x?=w277:bool)
        n105 = Compound Arithmetic op=AND(w278, w277) -> (w275:bool)
        n106 = Unbundle By Name(w297) -> ("Max Cell Voltage Actual Value"=w296:dbl, "Max Cell Voltage Derate Setpoint"=w298:dbl)
        n107 = Unbundle By Name(w307) -> ("Max Cell Voltage"=w293:sgl)
        n108 = local read "PV Breaker"() -> (w302:bool)
        n109 = call "Wait Timer.vi"("Boolean In"=w275, "Timer"=u32 5) -> ("Boolean Out"=w283:bool)  [unwired: 3 in]
        n110 = Greater Or Equal?(x=w293, y=sgl 4.1) -> (x >= y?=w288:bool)
        n111 = Less Or Equal?(x=w293, y=sgl 4.0) -> (x <= y?=w303:bool)
        n112 = Compound Arithmetic op=OR(w283, w288) -> (w287:bool)
        n113 = Compound Arithmetic op=OR(w303, w302) -> (w304:bool)
        n114 = call "RunAvg.vi"("Ignore avg?"=w276, "value in"=w296, "# of samples"=1000) -> ("value out"=w295:dbl)  [unwired: 4 in]
        n115 = Select(t=FALSE ("PV Breaker"), s=w287, f=w304) -> (s? t:f=w280:bool)
        n116 = Greater Or Equal?(x=w295, y=w298) -> (x >= y?=w281:bool)
        n117 = local write "PV Breaker"(w280) -> ()
        n118 = Compound Arithmetic op=AND(w280, w281) -> (w279:bool)
        n119 = call "PV Curtail Hz.vi"("1/I"=0.5, "PVCurtailEnable"=w279, "P"=0.015, "Error In"=w312, "reinitialize? (F)"=w276, "Current Limit Output"=w311, "FPGA Data"=w284) -> ("Error Out"=w291:errorcluster, "Frequency Setpoint"=w282:sgl)  [unwired: 3 in]
        n120 = Bundle By Name(cluster=w286, "Frequency SP"=w282) -> (w299:T4)
        n121 = Select(t=RT_State."SpotGen - Sync", s=w283, f=RT_State."SpotGen - Discharge") -> (s? t:f=w314:T12)
      }
      frame "SpotGen - Sync" {
        # "Disable HVAC"
        n122 = Equal?(x=w325, y=w324) -> (x = y?=w319:bool)
        n123 = Unbundle By Name(w323) -> ("PV Breaker Aux"=w321:bool)
        n124 = local read "HVAC CMD"() -> (w320:bool)
        n125 = Compound Arithmetic op=OR(w321, w320) -> (w317:bool)
        n126 = Not(x=w317) -> (.not. x?=w316:bool)
        n127 = And(x=w319, y=w316) -> (x .and. y?=w318:bool)
        n128 = call "Wait Timer.vi"("Boolean In"=w318, "Timer"=u32 60) -> ("Boolean Out"=w327:bool)  [unwired: 3 in]
        n129 = case shown="True" w327 {
          tunnel: w328 -> [w343 w346]
          tunnel: [w342 w345] -> w326
          frame False {
            n130 = Bundle By Name(cluster=w343, "Frequency SP"=sgl 60.0, "AC Current SP"=sgl 0.0) -> (w342:T4)
          }
          frame True {
            n131 = Bundle By Name(cluster=w346, "AC Voltage SP"=sgl 120.0 ("Voltage Setpoint"), "Op Mode SP"=MicroZed_Config_Op_Mode."Current Mode") -> (w345:T4)
          }
        }
        n132 = case shown="False" w317 {
          frame False {
            n133 = local write "Genset On"(TRUE ("Genset On")) -> ()
          }
          frame True {
          }
        }
        n134 = Unbundle By Name(w335) -> ("OP Mode FB"=w334:T5)
        n135 = local write "PV Breaker"(FALSE ("PV Breaker")) -> ()
        n136 = Equal?(x=w334, y=MicroZed_Config_Op_Mode."Current Mode") -> (x = y?=w333:bool)
        n137 = Select(t=RT_State."SpotGen - Charge", s=w333, f=RT_State."SpotGen - Sync") -> (s? t:f=w336:T12)
      }
      frame "Shutdown" {
        # "Power cycle power converter"
        n138 = Equal?(x=w371, y=w370) -> (x = y?=w348:bool)
        n139 = call "Wait Timer.vi"("Boolean In"=w348, "Timer"=u32 1) -> ("Boolean Out"=w349:bool)  [unwired: 3 in]
        n140 = Not(x=w349) -> (.not. x?=w350:bool)
        n141 = Bundle By Name(cluster=w357, "Op Mode SP"=MicroZed_Config_Op_Mode."Shutdown (Reset)") -> (w356:T4)
        n142 = local write "PC CMD"(w350) -> ()
        n143 = Not(x=w348) -> (.not. x?=w361:bool)
        n144 = call "Wait Timer.vi"("Boolean In"=w348, "Timer"=u32 3) -> ("Boolean Out"=w372:bool)  [unwired: 3 in]
        n145 = local write "Genset On"(TRUE ("Genset On")) -> ()
        n146 = call "Clear Faults.vi"("Initialize"=w361, "ES System Data"=w367, "PC Data"=w368, "FPGA Data"=w369, "Error In"=w355) -> ("Wait for Fault"=w359:bool, "Clear Error"=w353:bool, "Error Out"=w354:errorcluster)  [unwired: 8 in]
        n147 = case shown="True" w372 {
          tunnel: [RT_State."Shutdown" ("Real Time State") RT_State."Ready" ("Real Time State")] -> w363
          frame False {
          }
          frame True {
            n148 = local write "PV Breaker"(FALSE ("PV Breaker")) -> ()
            n149 = local write "SSG Breaker"(FALSE ("SSG Breaker")) -> ()
            n150 = local write "ES ON Array"(bool[] [FALSE, FALSE, FALSE, FALSE, FALSE, FALSE, FALSE, FALSE, FALSE, FALSE, FALSE] ("ES ON Array")) -> ()
          }
        }
        n151 = local write "Clear Error"(w353) -> ()
        n152 = local read "HVAC CMD"() -> (w358:bool)
        n153 = Not(x=w359) -> (.not. x?=w360:bool)
        n154 = Compound Arithmetic op=AND(w360, w358) -> (w362:bool)
        n155 = Select(t=w363, s=w362, f=RT_State."Shutdown" ("Real Time State")) -> (s? t:f=w366:T12)
      }
      frame "INVALID STATE" {
      }
    }
    n156 = Unbundle By Name(w119) -> ("E-Stop Aux"=w114:bool, "Overtemp Fault"=w113:bool, "Fire Fault"=w104:bool)
    n157 = Unbundle By Name(w122) -> ("PC Fault"=w116:bool, "PC Com Fault"=w115:bool)
    n158 = Unbundle By Name(w123) -> ("ES Fault"=w111:bool, "ES Com Fault"=w112:bool)
    n159 = Compound Arithmetic op=OR(w111, w112, w116, w115, w114, w113, w104) -> (w129:bool)
    n160 = Select(t=RT_State."Shutdown", s=w129, f=w131) -> (s? t:f=w121:T12)
    "Real Time State" <- w121
    n161 = Compound Arithmetic op=OR(w104, w102) -> (invert w103:bool)
    n162 = local write "PC Config"(w107) -> ()
    n163 = call "Wait Timer.vi"("Boolean In"=w103, "Timer"=u32 180) -> ("Boolean Out"=w110:bool)  [unwired: 3 in]
    n164 = Unbundle By Name(w105) -> ("status"=w126:bool)
    n165 = local read "stop"() -> (w127:bool)
    n166 = local write "HVAC CMD"(w110) -> ()
    n167 = Or(x=w126, y=w127) -> (x .or. y?=w128:bool)
  }
  n168 = while "FPGA Comms" {
    shift-right: [w384] -> w18
    shift-left: w44 -> [w399]
    tunnel: w43 -> [w398]
    tunnel: [w397] -> w19
    tunnel: w1 -> [w390]
    stop <- w400 stop-if-true
    # "IO controls via the cRIO FPGA"
    # "FPGA Comms"
    n169 = call "Watchdog Service.vi"("error in (no error)"=w399, "Watchdog Index"=w398) -> ("error out"=w391:errorcluster, "Watchdog Index Out"=w397:i32)  [unwired: 8 in]
    n170 = Wait Until Next ms Multiple(millisecond multiple=u32 50) -> ()  [unwired: 1 out]
    n171 = local read "PC CMD"() -> (w386:bool)
    n172 = local read "Generator ON West"() -> (w385:bool)
    n173 = local read "Generator ON East"() -> (w389:bool)
    n174 = local read "Real Time State"() -> (w388:T12)
    n175 = local read "HVAC CMD"() -> (w387:bool)
    n176 = call "FPGAData NightVision.vi"("FPGA VI Reference In"=w390, "SSG Breaker"="SSG Breaker", "PV Breaker"="PV Breaker", "Gen West On/Off"=w385, "Gen East On/Off"=w389, "Error In"=w391, "HVAC CMD"=w387, "PC CMD"=w386, "Real Time State"=w388) -> ("SSG Data Out"=→"FPGA Data":T9, "Automatic Start"=w393:bool, "HVAC FB"=→"HVAC FB":bool, "Error Out"=w384:errorcluster)  [unwired: 3 in]
    n177 = local write "Automatic Start"(w393) -> ()
    n178 = local read "stop"() -> (w400:bool)
  }
  n179 = while "Modbus Status Interface" {
    shift-right: [w415] -> w17
    shift-left: w40 -> [w418]
    tunnel: [w409] -> w16
    tunnel: w38 -> [w417]
    stop <- w420 stop-if-true
    # "Sends compiled data to the Host HMIs"
    # "Shared Variable to HMI"
    n180 = call "Watchdog Service.vi"("error in (no error)"=w418, "Watchdog Index"=w417) -> ("error out"=w416:errorcluster, "Watchdog Index Out"=w409:i32)  [unwired: 8 in]
    n181 = Wait Until Next ms Multiple(millisecond multiple=u32 200) -> ()  [unwired: 1 out]
    n182 = local read "Generator ON West"() -> (w404:bool)
    n183 = local read "Generator ON East"() -> (w403:bool)
    n184 = local read "Real Time State"() -> (w410:T12)
    n185 = local read "ES Cycle Count"() -> (w405:dbl)
    n186 = local read "ES System Data"() -> (w413:T10)
    n187 = local read "Gen Data West"() -> (w408:T2)
    n188 = local read "ES String Data"() -> (w414:T7)
    n189 = local read "Gen Data East"() -> (w407:T2)
    n190 = local read "FPGA Data"() -> (w411:T9)
    n191 = local read "PC Data"() -> (w412:T6)
    n192 = Build Array(w408, w407) -> (w406:T2[])
    n193 = Build Array(w404, w403) -> (w402:bool[])
    n194 = call "Modbus Status Interface.vi"("ES System Data In"=w413, "ES String Data"=w414, "Gen Data Array"=w406, "ES # Cycle Count"=w405, "PC Data In"=w412, "isGenOn"=w402, "FPGA Data In"=w411, "Error In"=w416, "Real Time State"=w410) -> ("Error Out"=w415:errorcluster)  [unwired: 6 in]
    n195 = local read "stop"() -> (w420:bool)
  }
  n196 = while "Generator Comms" {
    shift-right: [w421] -> w11
    shift-left: w12 -> [w430]
    tunnel: w10 -> [w428]
    tunnel: [w427] -> w9
    i -> [w424]
    stop <- w431 stop-if-true
    # "Modbus com to Gen West"
    # "Generator West Comms"
    n197 = call "Watchdog Service.vi"("error in (no error)"=w430, "Watchdog Index"=w428) -> ("error out"=w429:errorcluster, "Watchdog Index Out"=w427:i32)  [unwired: 8 in]
    n198 = Wait Until Next ms Multiple(millisecond multiple=u32 200 ("milliseconds to wait")) -> ()  [unwired: 1 out]
    n199 = call "ModbusComap.vi"("address"="192.168.50.215", "port (502)"=u16 502, "Unit ID"=u8 1, "Error In"=w429) -> ("Gen Data"=→"Gen Data West":T2, "Error Out"=w421:errorcluster)  [unwired: 5 in]
    n200 = local read "stop"() -> (w431:bool)
    "Gen West Count" <- w424
  }
  n201 = while "Generator Comms" {
    shift-right: [w433] -> w26
    shift-left: w27 -> [w442]
    tunnel: [w440] -> w25
    tunnel: w24 -> [w436]
    i -> [w437]
    stop <- w443 stop-if-true
    # "Modbus com to Gen East"
    # "Generator East Comms"
    n202 = call "Watchdog Service.vi"("error in (no error)"=w442, "Watchdog Index"=w436) -> ("error out"=w441:errorcluster, "Watchdog Index Out"=w440:i32)  [unwired: 8 in]
    n203 = Wait Until Next ms Multiple(millisecond multiple=u32 200 ("milliseconds to wait")) -> ()  [unwired: 1 out]
    n204 = call "ModbusComap.vi"("address"="192.168.50.216", "port (502)"=u16 502, "Unit ID"=u8 2, "Error In"=w441) -> ("Gen Data"=→"Gen Data East":T2, "Error Out"=w433:errorcluster)  [unwired: 5 in]
    n205 = local read "stop"() -> (w443:bool)
    "Gen East Count" <- w437
  }
  n206 = while "Generator Comms" {
    tunnel: w29 -> [_]
    stop <- w452 stop-if-true
    # "Logic to determine which \ngen to turn on"
    # "Generator Cycle"
    n207 = Wait Until Next ms Multiple(millisecond multiple=u32 200 ("milliseconds to wait")) -> ()  [unwired: 1 out]
    n208 = local read "Real Time State"() -> (w445:T12)
    n209 = local read "Gen Data West"() -> (w451:T2)
    n210 = local read "Gen Data East"() -> (w450:T2)
    n211 = call "Gen Cycle.vi"("Real Time State"=w445, "Gen East"=w450, "Gen West"=w451, "Generator ON"="Genset On") -> ("Gen Active"=→"Gen Active":T2, "Generator ON East"=→"Generator ON East":bool, "Generator ON West"=→"Generator ON West":bool)  [unwired: 5 in]
    n212 = local read "stop"() -> (w452:bool)
  }
  n213 = while "Power Converter Comms" {
    tunnel: w67 -> [w480]
    tunnel: [w478] -> w22
    shift-right: [w454] -> w23
    shift-left: w66 -> [w479]
    i -> [w461]
    stop <- w476 stop-if-true
    w455 = 208.0  # Current Limit
    # "PC coms. Also called\ninverter"
    # "Power Converter Comms"
    n214 = call "Watchdog Service.vi"("error in (no error)"=w479, "Watchdog Index"=w480) -> ("error out"=w475:errorcluster, "Watchdog Index Out"=w478:i32)  [unwired: 8 in]
    n215 = Wait Until Next ms Multiple(millisecond multiple=u32 100 ("milliseconds to wait")) -> ()  [unwired: 1 out]
    n216 = local read "Clear Error"() -> (w465:bool)
    n217 = local read "PC Config"() -> (w472:T4)
    n218 = local read "Current Limit Parameters"() -> (w460:T1)
    n219 = Unbundle By Name(w472) -> ("AC Current SP"=w473:sgl)
    n220 = local read "Real Time State"() -> (w456:T12)
    n221 = To Double Precision Float(number=w473) -> (double precision float=w469:dbl)
    n222 = Select(t="Manual OLP", s="Override?", f=w460) -> (s? t:f=w457:T1)
    n223 = call "Current Limit.vi"("Current Limit Parameters"=w457, "Current Limit"=w455, "Current In"=w469, "Real Time State"=w456, "Error In"=w475) -> ("Current Out"=w471:dbl, "Current Limit Output"=→"Current Limit Output":T3, "Error Out"=w474:errorcluster)  [unwired: 7 in, 1 out]
    n224 = Boolean To (0,1)(Boolean=w465) -> (0, 1=w466:i16)
    n225 = To Single Precision Float(number=w471) -> (single precision float=w468:sgl)
    n226 = Bundle By Name(cluster=w472, "Clear Faults SP"=w466, "AC Current SP"=w468) -> (w464:T4)
    n227 = call "Modbus MicroZed.vi"("Error In"=w474, "port (502)"=u16 1502, "address"="192.168.50.231", "PC Config"=w464) -> ("Error Out"=w454:errorcluster, "PC Data"=→"PC Data":T6)  [unwired: 6 in]
    n228 = local read "stop"() -> (w476:bool)
    "PC Count" <- w461
  }
  n229 = while "Energy Storage Comms" {
    shift-right: [w481] -> w15
    shift-left: w37 -> [w495]
    tunnel: w35 -> [w493]
    tunnel: [w488] -> w14
    i -> [w487]
    stop <- w497 stop-if-true
    # "Samsung Energy Storage\nAKA Batteries"
    # "Energy Storage Comms"
    n230 = call "Watchdog Service.vi"("error in (no error)"=w495, "Watchdog Index"=w493) -> ("error out"=w494:errorcluster, "Watchdog Index Out"=w488:i32)  [unwired: 8 in]
    n231 = Wait Until Next ms Multiple(millisecond multiple=u32 500 ("milliseconds to wait")) -> ()  [unwired: 1 out]
    n232 = local read "Clear Error"() -> (w485:bool)
    n233 = call "Modbus Samsung Mod.vi"("address"="192.168.50.246", "# Racks"=10, "port (502)"=u16 502, "Error In"=w494, "ES Reset"=w485, "ES ON Array"="ES ON Array") -> ("Error Out"=w481:errorcluster, "Current Limit Parameters Out"=→"Current Limit Parameters":T1, "Energy Storage String Data Out"=→"ES String Data":T7, "Energy Storage System Data Out"=→"ES System Data":T10, "Contactor CMD FB"=→"Contactor CMD FB":bool[])  [unwired: 1 in]
    n234 = local read "stop"() -> (w497:bool)
    "ES Count" <- w487
  }
  n235 = while "Check Watchdog" {
    tunnel: w1 -> [w498]
    shift-right: [w502] -> w60
    shift-left: w29 -> [w503]
    stop <- w501 stop-if-true
    w507 = u32 1000  # Max RT Loop Period (ms)
    # "Pets the FPGA. Otherwise it will go into a safe state"
    # "RT Watchdog"
    n236 = Wait Until Next ms Multiple(millisecond multiple=u32 100) -> ()  [unwired: 1 out]
    n237 = call "Watchdog Check.vi"("error in (no error)"=w503, "Timeout (ms)"=w507) -> ("error out"=w506:errorcluster, "Skipped?"=w509:bool, "Timeout?"=w508:bool)  [unwired: 6 in, 1 out]
    n238 = Compound Arithmetic op=AND(invert w508, invert w509) -> (w505:bool)
    n239 = xnode "Read/Write Control"("FPGA VI Reference In"=w498, "error in"=w506, "Pet RT Watchdog"=w505, "RT Safe"=TRUE) -> ("error out"=w502:errorcluster)  [unwired: 1 out]
    n240 = Unbundle By Name(w502) -> ("status"=w500:bool)
    n241 = local read "stop"() -> (w499:bool)
    n242 = Or(x=w500, y=w499) -> (x .or. y?=w501:bool)
  }
  n243 = call "Watchdog Disable.vi"("error in (no error)"=w17, "Watchdog Index"=w16) -> ("error out"=w45:errorcluster)  [unwired: 9 in]
  n244 = call "Watchdog Disable.vi"("error in (no error)"=w21, "Watchdog Index"=w20) -> ("error out"=w61:errorcluster)  [unwired: 9 in]
  n245 = call "Watchdog Disable.vi"("error in (no error)"=w18, "Watchdog Index"=w19) -> ("error out"=w31:errorcluster)  [unwired: 9 in]
  n246 = call "Watchdog Disable.vi"("error in (no error)"=w23, "Watchdog Index"=w22) -> ("error out"=w30:errorcluster)  [unwired: 9 in]
  n247 = call "Watchdog Disable.vi"("error in (no error)"=w15, "Watchdog Index"=w14) -> ("error out"=w32:errorcluster)  [unwired: 9 in]
  n248 = call "Watchdog Disable.vi"("error in (no error)"=w26, "Watchdog Index"=w25) -> ("error out"=w34:errorcluster)  [unwired: 9 in]
  n249 = call "Watchdog Disable.vi"("error in (no error)"=w11, "Watchdog Index"=w9) -> ("error out"=w33:errorcluster)  [unwired: 9 in]
  n250 = Merge Errors(w45, w60, w61, w31, w30, w32, w33, w34) -> (w69:errorcluster)
  n251 = xnode "Read/Write Control"("FPGA VI Reference In"=w1, "error in"=w69, "Enable RT Watchdog"=TRUE, "RT Safe"=FALSE ("Enable RT Watchdog")) -> ("FPGA VI Reference Out"=w71:refnum<k20>, "error out"=w70:errorcluster)
  n252 = xnode "Close FPGA VI Reference"("FPGA VI Reference In"=w71, "error in"=w70) -> ("error out"=w72:errorcluster)
  n253 = call <vilib>:"Clear Errors.vi"("error in (no error)"=w72) -> ()  [unwired: 5 in, 2 out]
